vi "solar_cfg Write File (Ref).vi"(0 "Config Path (*.ini)":path, 1 "Section (\"\" = Use Filename)":string, 2 "Comments (Key,Comment)":cluster{"Key":string, "Comment":string}[](array[cluster]), 5 "Key_Prefix (\"\")":string, 7 "Ctrl Refnums":refnum<vi>[](array[refnum]), 11 "error in (no error)":errorcluster, 12 "ArrayDelimiters (1D,2D)":string[](array[string])) -> (4 "Config Path out":path, 10 "Found?":bool, 15 "error out":errorcluster)   [LabVIEW 2018]
doc: "Write the values associated with a control reference to a specified section in the configuration file. If the Key is empty the control reference label is used instead. Set a Comment (#...) to add a description after the key's value. Clusters use the element lables are their key names. Set Enum as Strings to True to use the string item of an enum.\n\nSupported Data Types: \nI8..EXT, Enum, Boolean, String, Path, VISA Reference, Timestamp\n1D & 2D Arrays and Clusters of the data types above.\n\n[Section]\nKey = \"Value\" #Comment"
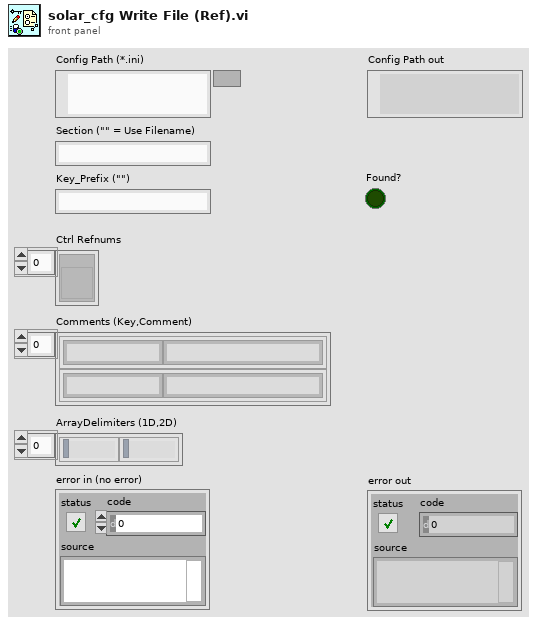
[diagram p1: front panel]
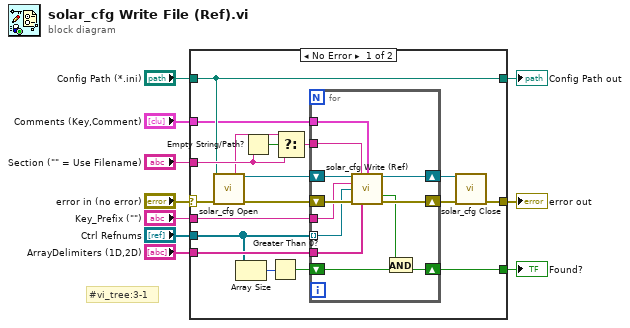
[diagram p0: block diagram]
diagram:
  # "#vi_tree:3-1"
  n1 = case shown="No Error" "error in (no error)" {
    selector: "error in (no error)" -> [w25 w42]
    tunnel: "Config Path (*.ini)" -> [w24 w41]
    tunnel: [w26 w42] -> w8
    tunnel: "Section (\"\" = Use Filename)" -> [w27 _]
    tunnel: [w24 w41] -> w6
    tunnel: "Ctrl Refnums" -> [w14 _]
    tunnel: "Key_Prefix (\"\")" -> [w16 _]
    tunnel: "Comments (Key,Comment)" -> [w19 _]
    tunnel: "ArrayDelimiters (1D,2D)" -> [w15 _]
    tunnel: [w11 _] -> w1
    frame No Error {
      n2 = call "solar_cfg Open.vi"("Config Path (*.ini)"=w24, "error in (no error)"=w25) -> ("Filename"=w23:string, "Config Refnum"=w21:refnum<data-value>, "error out"=w22:errorcluster)  [unwired: 10 in, 1 out]
      n3 = Array Size(array=w14) -> (size(s)=w13:i32)
      n4 = Empty String/Path?(string/path=w27) -> (empty?=w28:bool)
      n5 = Greater Than 0?(x=w13) -> (x > 0?=w12:bool)
      n6 = Select(t=w23, s=w28, f=w27) -> (s? t:f=w20:string)
      n7 = for {
        tunnel: w20 -> [w38]
        tunnel: w19 -> [w37]
        tunnel: w16 -> [w34]
        tunnel: w14 -> [w33] mode=indexing
        tunnel: w15 -> [w32]
        shift-right: [w35] -> w17
        shift-left: w22 -> [w40]
        shift-right: [w36] -> w18
        shift-left: w21 -> [w39]
        shift-right: [w29] -> w11
        shift-left: w12 -> [w31]
        n8 = call "solar_cfg Write (Ref).vi"("Config Refnum"=w39, "Section"=w38, "Comments (Key,Comment)"=w37, "Key_Prefix (\"\")"=w34, "Ctrl Refnum"=w33, "error in (no error)"=w40, "ArrayDelimiters (1D,2D)"=w32) -> ("dup Config Refnum"=w36:refnum<data-value>, "Found?"=w30:bool, "error out"=w35:errorcluster)  [unwired: 6 in]
        n9 = And(x=w30, y=w31) -> (x .and. y?=w29:bool)
      }
      n10 = call "solar_cfg Close.vi"("Config Refnum"=w18, "error in (no error)"=w17) -> ("error out"=w26:errorcluster)  [unwired: 12 in, 1 out]
    }
    frame Error {
    }
  }
  "error out" <- w8
  "Config Path out" <- w6
  "Found?" <- w1
